vi "Terminated.vi"(7 "Sender":refnum<class "Sender.lvclass">, 9 "Error":errorcluster, 10 "Actor":refnum<class "Actor.lvclass">) -> (2 "Msg":refnum<class "Msg.lvclass">)   [LabVIEW 2025, in "jettl.lvlib" / "Terminated Msg.lvlib"]
uses:
  Terminated Msg.lvlib
  Terminated Msg/Terminated Msg.lvclass
  C:/git/jettl/src/jettl/jettl/Terminated Msg/Has Destroyed Msg/Terminated Msg.lvclass
  C:/git/jettl/src/jettl/jettl/Msg/Msg.lvclass
  Msg/Msg.lvclass
  Actor/Actor/Actor.lvclass
  Sender/Sender/Sender.lvclass
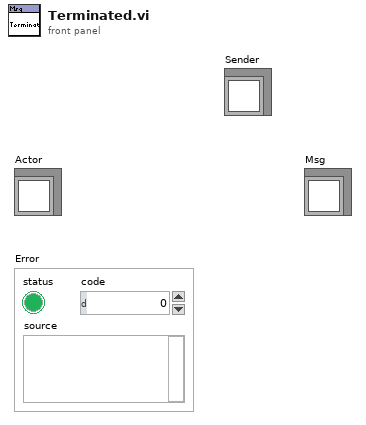
[diagram p1: front panel]
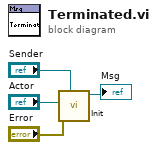
[diagram p0: block diagram]
diagram:
  n1 = call "Init.vi"("Sender"="Sender", "Error"="Error", "Actor"="Actor") -> ("Terminated Msg out"=→"Msg":refnum<class "Terminated Msg.lvclass">)  [unwired: 8 in]
